vi "ACKs_Control.vi"(8 "error in (no error)":errorcluster, 10 "ACK Q":refnum<queue>, 11 "SweepQ in":refnum<queue>) -> (0 "error out":errorcluster, 2 "Sweep Out":T1={"Temps(K)"=[], "Fields(T)"=[], "Sweep States"=enum."1. Idle", "PointStep"=enum."1. Scan_1", "Current Field"=0.0, "Current Temp"=0.0, "Expected_ACK"=enum."1. None", "ACK"=enum."1. None", "AfterAckStep"=enum."1. Idle", "Current Index Field"=0, "Current Index Temp"=0, "ACK Structure "=enum."Inner"}, 3 "SweepQ out":refnum<queue>)   [LabVIEW 2025]
uses:
  CTLS/Sweeper.ctl
  CTLS/ACK.ctl
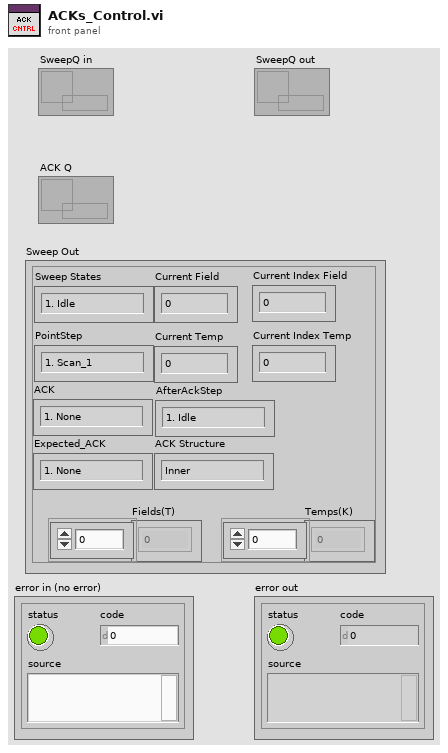
[diagram p1: front panel]
types:
  T1 = typedef "Sweeper.ctl" = cluster{"Temps(K)":dbl[], "Fields(T)":dbl[], "Sweep States":enum16{"1. Idle", "2. Start", "3. Apply_Config", "4. Run_Point_Step", "5. Wait ACK", "6. Next Field", "7. Next Temp", "8. Stop"}, "PointStep":enum16{"1. Init_Bias", "2. Init_Scan", "3. Field_Stable", "4. Temp_stable", "1. Scan_1", "2. DC_SF_1", "3. DC_BS_1", "4. Bias", "5. Scan_2", "6. DC_SF_2", "7. DC_BS_2", "8. Done"}, "Current Field":dbl, "Current Temp":dbl, "Expected_ACK":enum16{"1. None", "2. TempStable", "3. FieldStable", "4. ConfigApplied", "5. ScanDone", "6. BiasDone", "7. DriftDone (SF)", "8. DrifDone (BS)", "9. Done"}, "ACK":enum16{"1. None", "2. TempStable", "3. FieldStable", "4. ConfigApplied", "5. ScanDone", "6. BiasDone", "7. DriftDone (SF)", "8. DrifDone (BS)", "9. Done"}, "AfterAckStep":enum16{"1. Idle", "2. Start", "3. Apply_Config", "4. Run_Point_Step", "5. Wait ACK", "6. Next Field", "7. Next Temp", "8. Stop"}, "Current Index Field":i32, "Current Index Temp":i32, "ACK Structure ":enum16{"Inner", "Outer"}}
  T2 = typedef "ACK.ctl" = cluster{"ACK":enum16{"1. None", "2. TempStable", "3. FieldStable", "4. ConfigApplied", "5. ScanDone", "6. BiasDone", "7. DriftDone (SF)", "8. DrifDone (BS)"}}
  T3 = enum16{"1. None", "2. TempStable", "3. FieldStable", "4. ConfigApplied", "5. ScanDone", "6. BiasDone", "7. DriftDone (SF)", "8. DrifDone (BS)"}
  T4 = enum16{"1. Idle", "2. Start", "3. Stop", "4. Wait ACK", "5. Bias", "6. Scan", "7. Change Field", "8. Chang Temp", "9. Drift Correct (SF)", "10. Drift Correct (BS)", "11. Next Field", "12. Next Temp"}
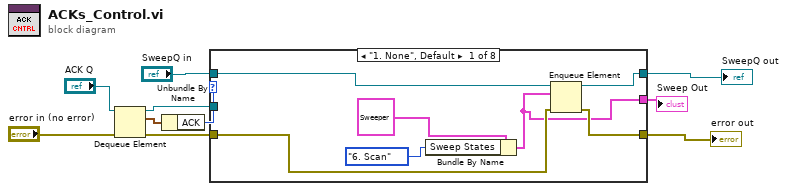
[diagram p0: block diagram]
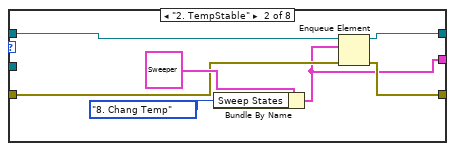
[diagram p2: hidden frame]
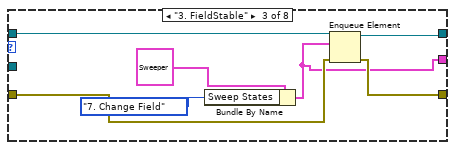
[diagram p3: hidden frame]
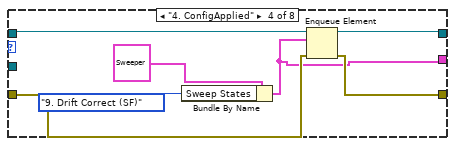
[diagram p4: hidden frame]
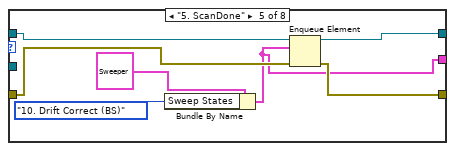
[diagram p5: hidden frame]
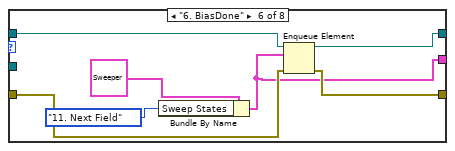
[diagram p6: hidden frame]
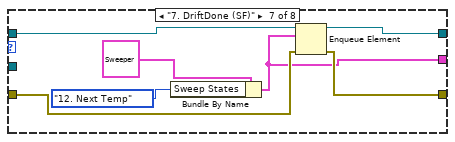
[diagram p7: hidden frame]
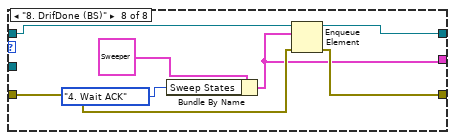
[diagram p8: hidden frame]
diagram:
  n1 = Dequeue Element(queue="ACK Q", error in (no error)="error in (no error)") -> (queue out=w5:refnum<queue>, element=w3:T2, error out=w6:errorcluster)  [unwired: 1 in, 1 out]
  n2 = Unbundle By Name(w3) -> ("ACK"=w4:T3)
  n3 = case shown="\"1. None\", Default" w4 {
    tunnel: w5 -> [_ _ _ _ _ _ _ _]
    tunnel: w6 -> [w12 w21 w29 w33 w42 w50 w54 w63]
    tunnel: "SweepQ in" -> [w17 w22 w27 w36 w41 w51 w58 w62]
    tunnel: [w14 w20 w26 w35 w40 w48 w56 w61] -> w9
    tunnel: [w13 w19 w30 w34 w43 w49 w57 w64] -> w10
    tunnel: [w11 w18 w25 w32 w39 w46 w53 w60] -> w1
    frame "1. None", Default {
      n4 = Bundle By Name(cluster=T1 {"Temps(K)"=[], "Fields(T)"=[], "Sweep States"=enum."1. Idle", "PointStep"=enum."1. Scan_1", "Current Field"=0.0, "Current Temp"=0.0, "Expected_ACK"=enum."1. None", "ACK"=enum."1. None", "AfterAckStep"=enum."1. Idle", "Current Index Field"=0, "Current Index Temp"=0, "ACK Structure "=enum."Inner"} ("Temp and Field Range"), "Sweep States"=T4."6. Scan") -> (w11:T1)
      n5 = Enqueue Element(queue=w17, element=w11, error in (no error)=w12) -> (queue out=w14:refnum<queue>, error out=w13:errorcluster)  [unwired: 1 in, 1 out]
    }
    frame "2. TempStable" {
      n6 = Bundle By Name(cluster=T1 {"Temps(K)"=[], "Fields(T)"=[], "Sweep States"=enum."1. Idle", "PointStep"=enum."1. Scan_1", "Current Field"=0.0, "Current Temp"=0.0, "Expected_ACK"=enum."1. None", "ACK"=enum."1. None", "AfterAckStep"=enum."1. Idle", "Current Index Field"=0, "Current Index Temp"=0, "ACK Structure "=enum."Inner"} ("Temp and Field Range"), "Sweep States"=T4."8. Chang Temp") -> (w18:T1)
      n7 = Enqueue Element(queue=w22, element=w18, error in (no error)=w21) -> (queue out=w20:refnum<queue>, error out=w19:errorcluster)  [unwired: 1 in, 1 out]
    }
    frame "3. FieldStable" {
      n8 = Bundle By Name(cluster=T1 {"Temps(K)"=[], "Fields(T)"=[], "Sweep States"=enum."1. Idle", "PointStep"=enum."1. Scan_1", "Current Field"=0.0, "Current Temp"=0.0, "Expected_ACK"=enum."1. None", "ACK"=enum."1. None", "AfterAckStep"=enum."1. Idle", "Current Index Field"=0, "Current Index Temp"=0, "ACK Structure "=enum."Inner"} ("Temp and Field Range"), "Sweep States"=T4."7. Change Field") -> (w25:T1)
      n9 = Enqueue Element(queue=w27, element=w25, error in (no error)=w29) -> (queue out=w26:refnum<queue>, error out=w30:errorcluster)  [unwired: 1 in, 1 out]
    }
    frame "4. ConfigApplied" {
      n10 = Bundle By Name(cluster=T1 {"Temps(K)"=[], "Fields(T)"=[], "Sweep States"=enum."1. Idle", "PointStep"=enum."1. Scan_1", "Current Field"=0.0, "Current Temp"=0.0, "Expected_ACK"=enum."1. None", "ACK"=enum."1. None", "AfterAckStep"=enum."1. Idle", "Current Index Field"=0, "Current Index Temp"=0, "ACK Structure "=enum."Inner"} ("Temp and Field Range"), "Sweep States"=T4."9. Drift Correct (SF)") -> (w32:T1)
      n11 = Enqueue Element(queue=w36, element=w32, error in (no error)=w33) -> (queue out=w35:refnum<queue>, error out=w34:errorcluster)  [unwired: 1 in, 1 out]
    }
    frame "5. ScanDone" {
      n12 = Bundle By Name(cluster=T1 {"Temps(K)"=[], "Fields(T)"=[], "Sweep States"=enum."1. Idle", "PointStep"=enum."1. Scan_1", "Current Field"=0.0, "Current Temp"=0.0, "Expected_ACK"=enum."1. None", "ACK"=enum."1. None", "AfterAckStep"=enum."1. Idle", "Current Index Field"=0, "Current Index Temp"=0, "ACK Structure "=enum."Inner"} ("Temp and Field Range"), "Sweep States"=T4."10. Drift Correct (BS)") -> (w39:T1)
      n13 = Enqueue Element(queue=w41, element=w39, error in (no error)=w42) -> (queue out=w40:refnum<queue>, error out=w43:errorcluster)  [unwired: 1 in, 1 out]
    }
    frame "6. BiasDone" {
      n14 = Bundle By Name(cluster=T1 {"Temps(K)"=[], "Fields(T)"=[], "Sweep States"=enum."1. Idle", "PointStep"=enum."1. Scan_1", "Current Field"=0.0, "Current Temp"=0.0, "Expected_ACK"=enum."1. None", "ACK"=enum."1. None", "AfterAckStep"=enum."1. Idle", "Current Index Field"=0, "Current Index Temp"=0, "ACK Structure "=enum."Inner"} ("Temp and Field Range"), "Sweep States"=T4."11. Next Field") -> (w46:T1)
      n15 = Enqueue Element(queue=w51, element=w46, error in (no error)=w50) -> (queue out=w48:refnum<queue>, error out=w49:errorcluster)  [unwired: 1 in, 1 out]
    }
    frame "7. DriftDone (SF)" {
      n16 = Bundle By Name(cluster=T1 {"Temps(K)"=[], "Fields(T)"=[], "Sweep States"=enum."1. Idle", "PointStep"=enum."1. Scan_1", "Current Field"=0.0, "Current Temp"=0.0, "Expected_ACK"=enum."1. None", "ACK"=enum."1. None", "AfterAckStep"=enum."1. Idle", "Current Index Field"=0, "Current Index Temp"=0, "ACK Structure "=enum."Inner"} ("Temp and Field Range"), "Sweep States"=T4."12. Next Temp") -> (w53:T1)
      n17 = Enqueue Element(queue=w58, element=w53, error in (no error)=w54) -> (queue out=w56:refnum<queue>, error out=w57:errorcluster)  [unwired: 1 in, 1 out]
    }
    frame "8. DrifDone (BS)" {
      n18 = Bundle By Name(cluster=T1 {"Temps(K)"=[], "Fields(T)"=[], "Sweep States"=enum."1. Idle", "PointStep"=enum."1. Scan_1", "Current Field"=0.0, "Current Temp"=0.0, "Expected_ACK"=enum."1. None", "ACK"=enum."1. None", "AfterAckStep"=enum."1. Idle", "Current Index Field"=0, "Current Index Temp"=0, "ACK Structure "=enum."Inner"} ("Temp and Field Range"), "Sweep States"=T4."4. Wait ACK") -> (w60:T1)
      n19 = Enqueue Element(queue=w62, element=w60, error in (no error)=w63) -> (queue out=w61:refnum<queue>, error out=w64:errorcluster)  [unwired: 1 in, 1 out]
    }
  }
  "error out" <- w10
  "SweepQ out" <- w9
  "Sweep Out" <- w1
